vi "Init.vi"(4 "Application Ref":refnum<vi>, 5 "Alias":string, 6 "Actor Ref":refnum<vi>, 7 "Address":refnum<user-event>, 9 "Unified Msg Set":T1, 10 "Event Ref":refnum<event-registration>) -> (3 "Base Attributes out":refnum<class "Base Attributes.lvclass">)   [LabVIEW 2020, in "jettl.lvlib" / "Attributes.lvlib" / "Base Attributes.lvclass"]
uses:
  Base Attributes.lvclass
  Msg/Msg.lvclass
  Actor/Msg Set.ctl
  Base Attributes.lvclass/Base Attributes.ctl
  Actor/Actor.lvlib
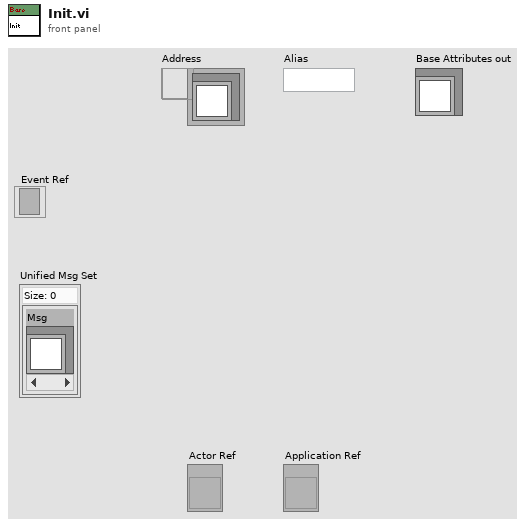
[diagram p1: front panel]
types:
  T1 = typedef "jettl.lvlib/Actor.lvlib/Msg Set.ctl" = set{refnum<class "Msg.lvclass">}
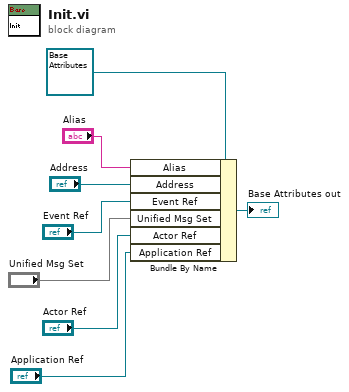
[diagram p0: block diagram]
diagram:
  n1 = Bundle By Name(cluster=refnum<class "Base Attributes.lvclass"> refnum ("Base Attributes in"), "Alias"="Alias", "Address"="Address", "Event Ref"="Event Ref", "Unified Msg Set"="Unified Msg Set", "Actor Ref"="Actor Ref", "Application Ref"="Application Ref") -> (→"Base Attributes out":refnum<class "Base Attributes.lvclass">)
